vi "Write Strg.vi"(8 "error in (no error)":errorcluster, 10 "Strg":string, 11 "ClassData in":refnum<class "ClassData.lvclass">) -> (0 "error out":errorcluster, 3 "ClassData out":refnum<class "ClassData.lvclass">)   [LabVIEW 2018, in "ClassData.lvclass"]
uses:
  ClassData.lvclass
  ClassData.lvclass/ClassData.ctl
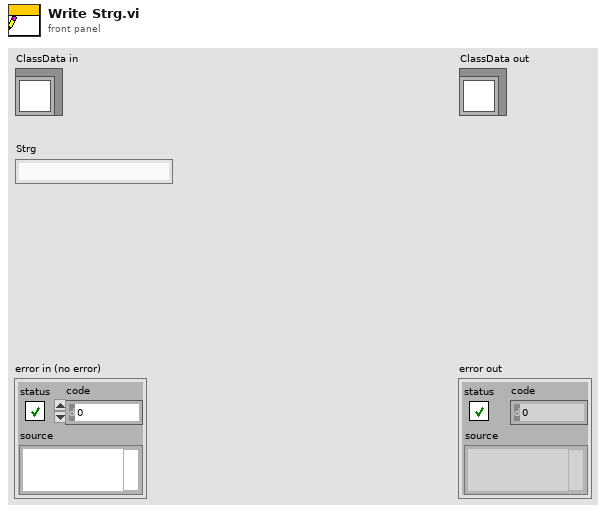
[diagram p1: front panel]
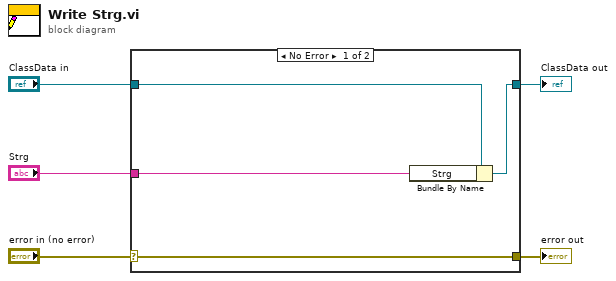
[diagram p0: block diagram]
diagram:
  n1 = case shown="No Error" "error in (no error)" {
    selector: "error in (no error)" -> [w9 w10]
    tunnel: [w9 w10] -> w4
    tunnel: [w7 w11] -> w2
    tunnel: "ClassData in" -> [w8 w11]
    tunnel: "Strg" -> [w6 _]
    frame No Error {
      n2 = Bundle By Name(cluster=w8, "Strg"=w6) -> (w7:refnum<class "ClassData.lvclass">)
    }
    frame Error {
    }
  }
  "error out" <- w4
  "ClassData out" <- w2
